vi "Look up nested object.vi"(8 "error in (no error)":errorcluster, 9 "Supress  dialog":bool, 10 "Object name":string, 11 "Mag Lab Measure Base in":refnum<class "Mag Lab Measure Base.lvclass">) -> (0 "error out":errorcluster, 1 "Object Queue":refnum<class "Message Enqueuer.lvclass">, 2 "Found?":bool, 3 "Mag Lab Measure Base out":refnum<class "Mag Lab Measure Base.lvclass">)   [LabVIEW 2015, in "Mag Lab Measure Base.lvclass"]
uses:
  Mag Lab Measure Base.lvclass
  <vilib>/ActorFramework/Message Enqueuer/Message Enqueuer.lvclass
  Mag Lab Root/Mag Lab Root.lvclass/Mag Lab Root.ctl
  Mag Lab Measure Base.lvclass/Mag Lab Measure Base.ctl
  <vilib>/ActorFramework/Actor/Actor.lvclass/Actor.ctl
  <vilib>/ActorFramework/Message Enqueuer/Message Enqueuer.lvclass/Message Enqueuer.ctl
  <vilib>/ActorFramework/Message Enqueuer/Init from Existing Queue.vi
  <vilib>/ActorFramework/Actor/Actor.lvclass
  Mag Lab Root/Mag Lab Root.lvclass
panel:
  in  "Self Enqueuer":refnum<class "Message Enqueuer.lvclass">
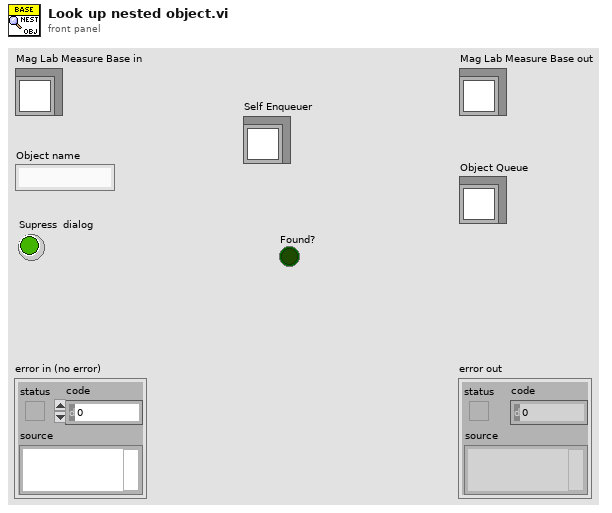
[diagram p1: front panel]
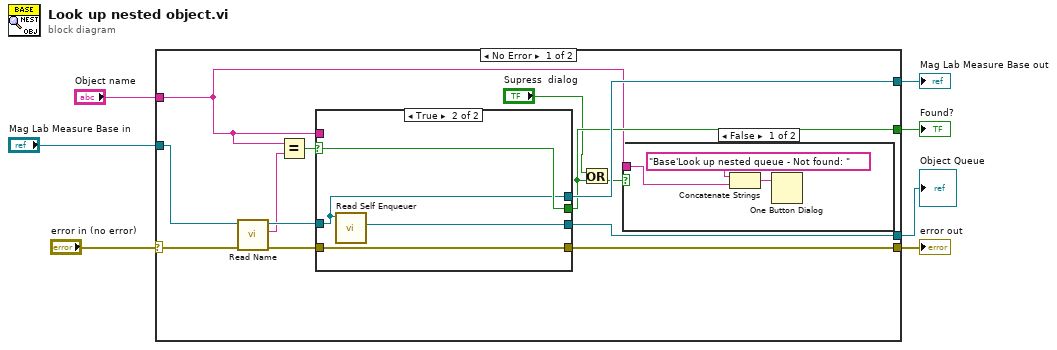
[diagram p0: block diagram]
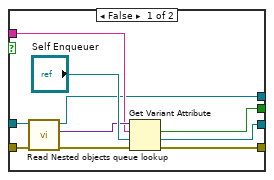
[diagram p2: hidden frame]
diagram:
  n1 = case shown="No Error" "error in (no error)" {
    selector: "error in (no error)" -> [w11 w39]
    tunnel: [w19 w39] -> w6
    tunnel: [w18 w38] -> w4
    tunnel: "Mag Lab Measure Base in" -> [w10 w38]
    tunnel: "Object name" -> [w16 _]
    tunnel: [w20 _] -> w2
    tunnel: [w17 _] -> w1
    frame No Error {
      n2 = call "Read Name.vi"("error in (no error)"=w11, "Mag Lab Root in"=w10) -> ("error out"=w12:errorcluster, "Name"=w13:string, "Mag Lab Root out"=w14:refnum<class "Mag Lab Measure Base.lvclass">)  [unwired: 7 in]
      n3 = Equal?(x=w16, y=w13) -> (x = y?=w15:bool)
      n4 = case shown="True" w15 {
        selector: w15 -> [_ w32]
        tunnel: w14 -> [w30 w31]
        tunnel: [w27 w34] -> w20
        tunnel: w12 -> [w26 w33]
        tunnel: [w25 w33] -> w19
        tunnel: [w21 w32] -> w17
        tunnel: [w22 w31] -> w18
        tunnel: w16 -> [w24 _]
        frame False {
          n5 = call "Read Nested objects queue lookup.vi"("error in (no error)"=w26, "Mag Lab Measure Base in"=w30) -> ("error out"=w23:errorcluster, "Nested objects queue lookup"=w28:variant, "Mag Lab Measure Base out"=w22:refnum<class "Mag Lab Measure Base.lvclass">)  [unwired: 7 in]
          n6 = Get Variant Attribute(Variant=w28, name=w24, default value (empty Variant)="Self Enqueuer", error in=w23) -> (found=w21:bool, value=w27:refnum<class "Message Enqueuer.lvclass">, error out=w25:errorcluster)  [unwired: 1 out]
        }
        frame True {
          n7 = call <vilib>:"Read Self Enqueuer.vi"("Actor"=w31) -> ("Self Enqueuer"=w34:refnum<class "Message Enqueuer.lvclass">)  [unwired: 10 in]
        }
      }
      n8 = Or(x="Supress  dialog", y=w17) -> (x .or. y?=w9:bool)
      n9 = case shown="False" w9 {
        tunnel: w16 -> [w35 _]
        frame False {
          n10 = Concatenate Strings("Base'Look up nested queue - Not found: ", w35) -> (w36:string)
          n11 = One Button Dialog(message=w36) -> ()  [unwired: 1 in, 1 out]
        }
        frame True {
        }
      }
    }
    frame Error {
    }
  }
  "error out" <- w6
  "Mag Lab Measure Base out" <- w4
  "Object Queue" <- w2
  "Found?" <- w1
